vi "DisconnectHardware.vi"(8 "Error In":errorcluster, 11 "MainData":T1) -> (0 "Error Out":errorcluster, 3 "MainData out":T1)   [LabVIEW 2019, in "MainController.lvlib"]
uses:
  MainController.lvlib
  Cluster - MainData.ctl
  All Message Queues.ctl
  Cluster - MainControllerMessage.ctl
  Enum - MainState.ctl
  AutoMode/Cluster - AutoModeMessage.ctl
  AutoMode/Enum - AutoModeState.ctl
  ManualMode/Cluster - ManualModeMessageCluster.ctl
  ManualMode/Enum - ManualModeMessage.ctl
  Settings/CTL_MessageCluster.ctl
  Settings/CTL_SettingsMessage.ctl
  Cluster - HardwareConfiguration.ctl
  Cluster - LoggingConfiguration.ctl
  Cluster - TestSettings.ctl
  UI State.ctl
  UI Data.ctl
  Mark10 API/Mark 10 TSTM-DC.lvlib
  AutoMode/AutoMode.lvlib
  ManualMode/ManualMode.lvlib
  Settings/Settings.lvlib
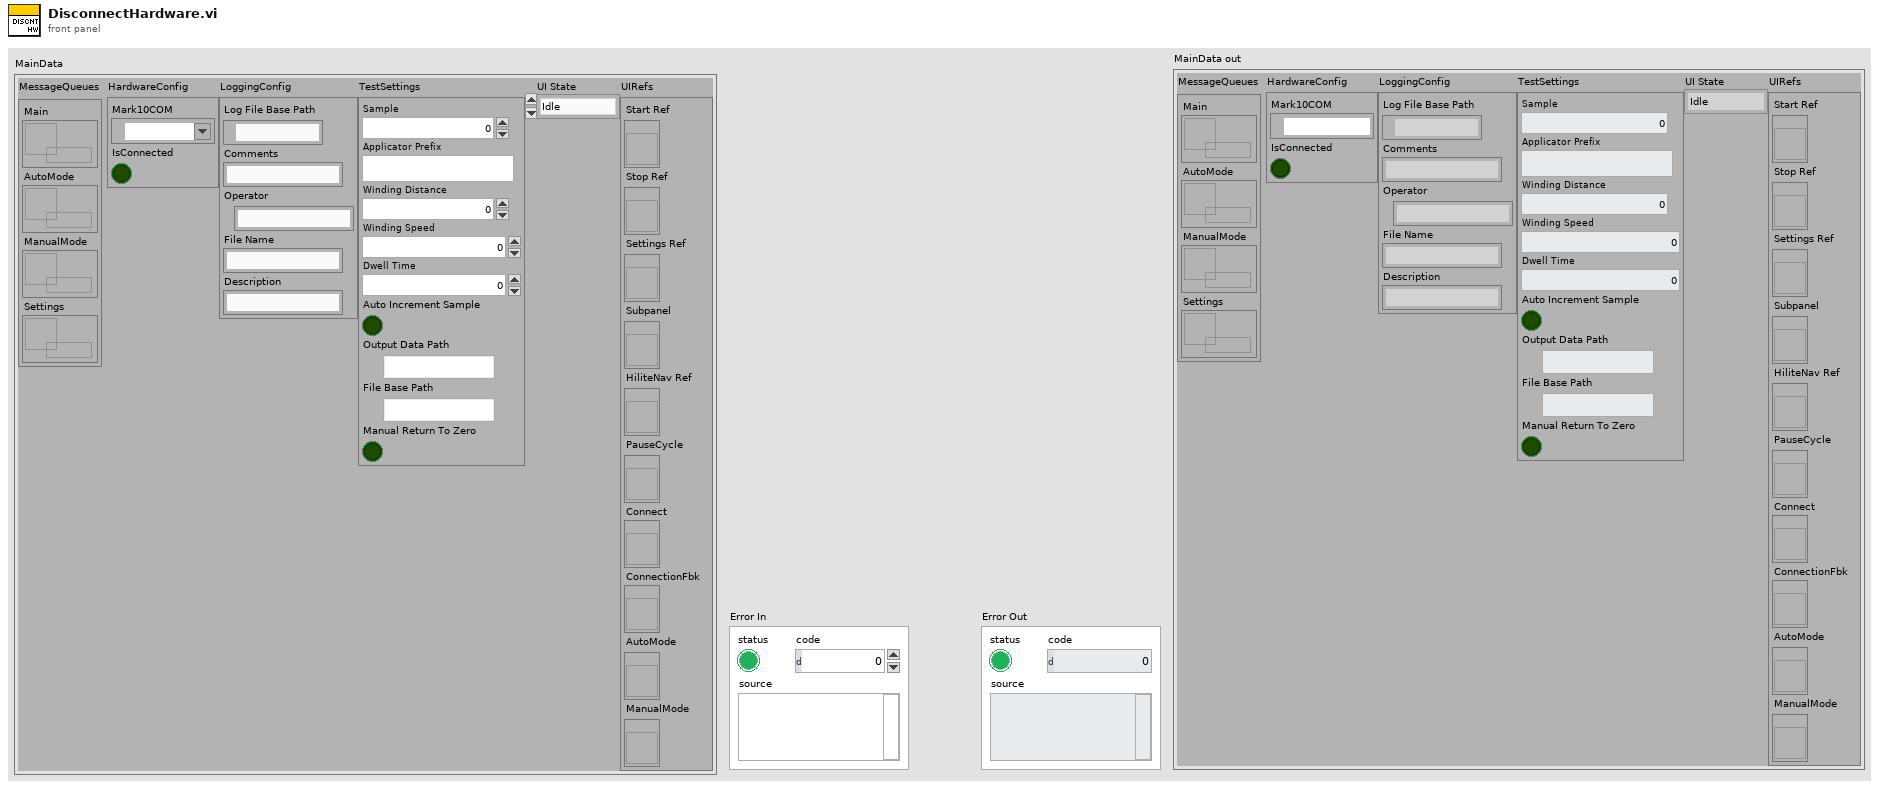
[diagram p1: front panel]
types:
  T1 = typedef "MainController.lvlib/Cluster - MainData.ctl" = cluster{"MessageQueues":T2, "HardwareConfig":T3, "LoggingConfig":T4, "TestSettings":T5, "UI State":T6, "UIRefs":T7}
  T2 = typedef "MainController.lvlib/All Message Queues.ctl" = cluster{"Main":refnum<queue>, "AutoMode":refnum<queue>, "ManualMode":refnum<queue>, "Settings":refnum<queue>}
  T3 = typedef "MainController.lvlib/Cluster - HardwareConfiguration.ctl" = cluster{"Mark10COM":refnum<visa-resource-name>, "IsConnected":bool}
  T4 = typedef "MainController.lvlib/Cluster - LoggingConfiguration.ctl" = cluster{"Log File Base Path":path, "Comments ":string, "Operator":string, "File Name":string, "Description":string}
  T5 = typedef "MainController.lvlib/Cluster - TestSettings.ctl" = cluster{"Sample":u32, "Applicator Prefix":string, "Winding Distance":dbl, "Winding Speed":dbl, "Dwell Time":dbl, "Auto Increment Sample":bool, "Output Data Path":path, "File Base Path":path, "Manual Return To Zero":bool}
  T6 = typedef "MainController.lvlib/UI State.ctl" = enum16{"Idle", "AutoIdle", "AutoRunning", "ManualMode", "Settings"}
  T7 = typedef "MainController.lvlib/UI Data.ctl" = cluster{"Start Ref":refnum<vi>, "Stop Ref":refnum<vi>, "Settings Ref":refnum<vi>, "Subpanel":refnum<vi>, "HiliteNav Ref":refnum<vi>, "PauseCycle":refnum<vi>, "Connect":refnum<vi>, "ConnectionFbk":refnum<vi>, "AutoMode":refnum<vi>, "ManualMode":refnum<vi>}
  T8 = typedef "MainController.lvlib/Enum - MainState.ctl" = enum16{"Initialize", "InitUIRefs", "LaunchSettings", "LaunchAutoMode", "LaunchManualMode", "LaunchTestReport", "ConnectHardware", "DisconnectHardware", "HiliteNavItems", "StartAutoMode", "PauseAutoMode", "StopAutoMode", "ShowFlyout", "HideFlyout", "BroadcastSettings", "PickupTestSettings", "BroadcastHW", "AutoTestDone", "DAQStatus", "UpdateCommandBar", "Error", "RecieveError", "Exit"}
  T9 = typedef "AutoMode.lvlib/Enum - AutoModeState.ctl" = enum16{"Initialize", "Idle", "UpdateConfig", "UpdateHWConfig", "BroadcastSettings", "Start", "CheckValidReportPath", "Winding", "WaitForWinding", "Unwind", "WaitForUnwind", "Stop", "Abort", "WriteDataToFile", "EventTriggered", "GenerateFilePath", "ZeroPosition", "GotoZero", "Error", "Exit"}
  T10 = typedef "ManualMode.lvlib/Enum - ManualModeMessage.ctl" = enum16{"Initialize", "Idle", "Start", "Stop", "Pause", "Resume", "BroadcastPreCollection", "MoveCCW", "MoveCW", "StopMove", "SetZero", "GotoZero", "UpdateHW", "SendMark10Cmd", "ReadPosition", "ReadTorque", "ReadStatus", "Error", "Exit"}
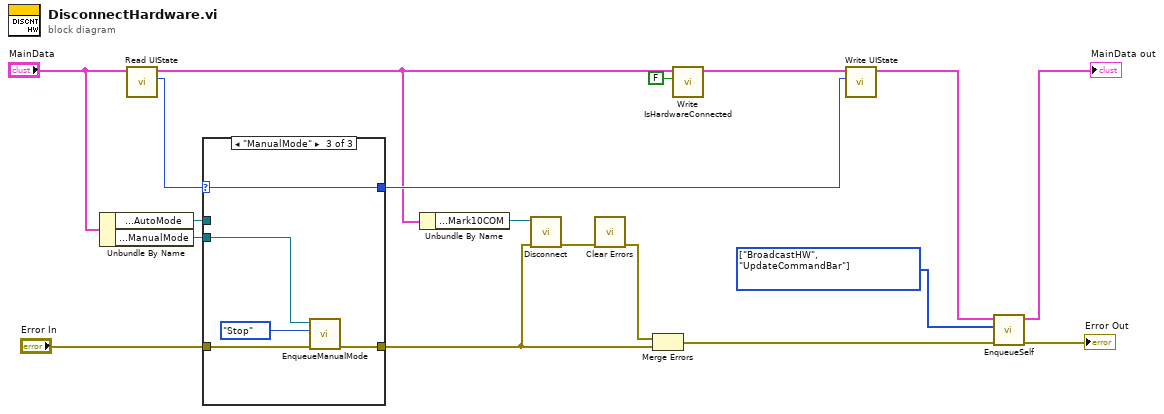
[diagram p0: block diagram]
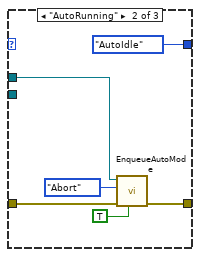
[diagram p3: hidden frame]
diagram:
  w1 = T8[] [enum."BroadcastHW", enum."UpdateCommandBar"] items=["Initialize", "InitUIRefs", "LaunchSettings", "LaunchAutoMode", "LaunchManualMode", "LaunchTestReport", "ConnectHardware", "DisconnectHardware", "HiliteNavItems", "StartAutoMode", "PauseAutoMode", "StopAutoMode", "ShowFlyout", "HideFlyout", "BroadcastSettings", "PickupTestSettings", "BroadcastHW", "AutoTestDone", "DAQStatus", "UpdateCommandBar", "Error", "RecieveError", "Exit"] ("Message")
  n1 = Unbundle By Name("MainData") -> ("MessageQueues.AutoMode"=w18:refnum<queue>, "MessageQueues.ManualMode"=w14:refnum<queue>)
  n2 = call "Read UIState.vi"("MainData"="MainData") -> ("UI State"=w8:T6, "MainData out"=w6:T1)  [unwired: 9 in]
  n3 = case shown="\"ManualMode\"" w8 {
    selector: w8 -> [w20 _ w30]
    tunnel: [w20 UI_State."AutoIdle" ("UI State") w30] -> w10
    tunnel: "Error In" -> [w19 w25 w31]
    tunnel: [w19 w24 w29] -> w15
    tunnel: w18 -> [_ w23 _]
    tunnel: w14 -> [_ _ w28]
    frame "Idle", Default {
    }
    frame "AutoRunning" {
      n4 = call "EnqueueAutoMode.vi"("Priority Message"=TRUE, "error in (no error)"=w25, "AutoState"=Enum_-_AutoModeState."Abort" ("CycleTestState"), "Queue in"=w23) -> ("error out"=w24:errorcluster)  [unwired: 6 in, 1 out]
    }
    frame "ManualMode" {
      n5 = call "EnqueueManualMode.vi"("error in (no error)"=w31, "Message"=Enum_-_ManualModeMessage."Stop", "queue"=w28) -> ("error out"=w29:errorcluster)  [unwired: 7 in, 1 out]
    }
  }
  n6 = Unbundle By Name(w6) -> ("HardwareConfig.Mark10COM"=w16:refnum<visa-resource-name>)
  n7 = call "Disconnect.vi"("error in (no error)"=w15, "VISA resource name"=w16) -> ("error out"=w17:errorcluster)  [unwired: 8 in, 1 out]
  n8 = call <vilib>:"Clear Errors.vi"("error in (no error)"=w17) -> ("error out"=w13:errorcluster)  [unwired: 5 in, 1 out]
  n9 = Merge Errors(w13, w15) -> (w12:errorcluster)
  n10 = call "Write IsHardwareConnected.vi"("HardwareConfig.IsConnected"=FALSE, "MainData in"=w6) -> ("MainData out 2"=w11:T1)  [unwired: 9 in]
  n11 = call "Write UIState.vi"("UI State"=w10, "MainData"=w11) -> ("MainData out"=w3:T1)  [unwired: 9 in]
  n12 = call "EnqueueSelf.vi"("Error In"=w12, "Messages"=w1, "MainData"=w3) -> ("Error Out"=→"Error Out":errorcluster, "MainData out"=→"MainData out":T1)  [unwired: 7 in]
